vi "output.vi"(8 "error in":errorcluster, 10 "data table in":T1, 11 "Shared Library Module runtime in":refnum<class "Shared Library Module runtime.lvclass">) -> (0 "error out":errorcluster, 2 "data table out":T1, 3 "Shared Library Module runtime out":refnum<class "Shared Library Module runtime.lvclass">)   [LabVIEW 2013, in "Shared Library Module runtime.lvclass"]
doc: "Provides an interface for writing data to a module at runtime. While this interface performs no operations, a child should provide an override which may write to any open sessions, references, or interfaces.Platypus Framework 1.0.1.60\nNI Systems Engineering - National Instruments"
uses:
  Shared Library Module runtime.lvclass
  <vilib>/NI/Tag Bus/table/data table.ctl
  Shared Library Module runtime.lvclass/Shared Library Module runtime.ctl
  <vilib>/NI/Tag Bus/table/data table.lvlib
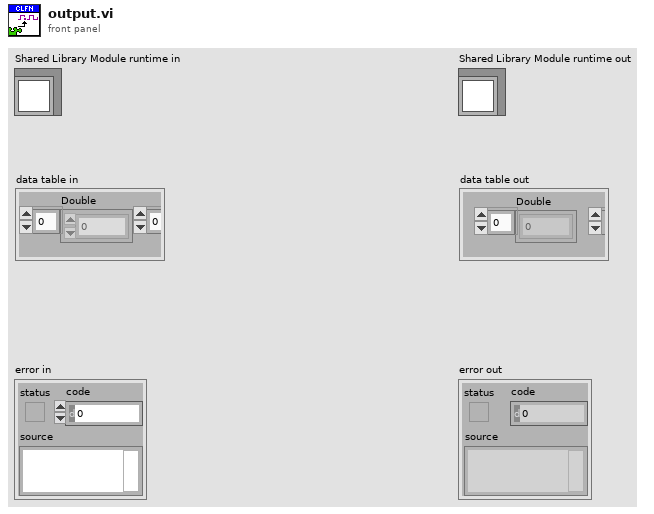
[diagram p1: front panel]
types:
  T1 = typedef "tag bus.lvlib/data table.lvlib/data table.ctl" = cluster{"Double":dbl[], "Single":sgl[], "I64":i64[], "I32":i32[], "I16":i16[], "I8":i8[], "U64":u64[], "U32":u32[], "U16":u16[], "U8":u8[], "Boolean":bool[], "String":string[], "Array of Double":cluster{"DBL Array":dbl[]}[], "Array of Single":cluster{"SGL Array":sgl[]}[], "Array of I64":cluster{"I64 Array":i64[]}[], "Array of I32":cluster{"I32 Array":i32[]}[], "Array of I16":cluster{"I16 Array":i16[]}[], "Array of I8":cluster{"I8 Array":i8[]}[], "Array of U64":cluster{"U64 Array":u64[]}[], "Array of U32":cluster{"U32 Array":u32[]}[], "Array of U16":cluster{"U16 Array":u16[]}[], "Array of U8":cluster{"U8 Array":u8[]}[], "Array of Boolean":cluster{"Boolean Array":bool[]}[], "Array of String":cluster{"String Array":string[]}[]}
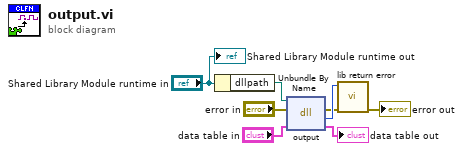
[diagram p0: block diagram]
diagram:
  n1 = Unbundle By Name("Shared Library Module runtime in") -> ("dllpath"=w8:path)
  n2 = dll-call lib="?" fn="output"(path in=w8, error in="error in", "lvdataclusterin"="data table in") -> (error out=w2:errorcluster, "return type"=w3:i32, "lvdataclusterin"=→"data table out":T1)  [unwired: 1 in, 1 out]
  n3 = call "lib return error.vi"("error in"=w2, "return value"=w3) -> ("error out"=→"error out":errorcluster)  [unwired: 9 in]
  "Shared Library Module runtime out" <- "Shared Library Module runtime in"
